vi "LED flashing 2.vi"(0 "Arduino Resource In":T1={"VISA resource"="", "Board Type"=enum."Uno", "Connection Type"=enum."USB / Serial", "Bytes Per Packet (15)"=15}, 11 "Error In":errorcluster, 12 "Текущий раствор":i32) -> (1 "1":bool, 2 "2":bool, 3 "3":bool, 4 "Arduino Resource Out":T1={"VISA resource"="", "Board Type"=enum."Uno", "Connection Type"=enum."USB / Serial", "Bytes Per Packet (15)"=15}, 15 "Error Out":errorcluster)   [LabVIEW 2016]
uses:
  <vilib>/LabVIEW Interface for Arduino/Type Defs/Arduino Resource.ctl
  <vilib>/LabVIEW Interface for Arduino/Type Defs/Board Type.ctl
  <vilib>/LabVIEW Interface for Arduino/LabVIEW Interface for Arduino.lvlib
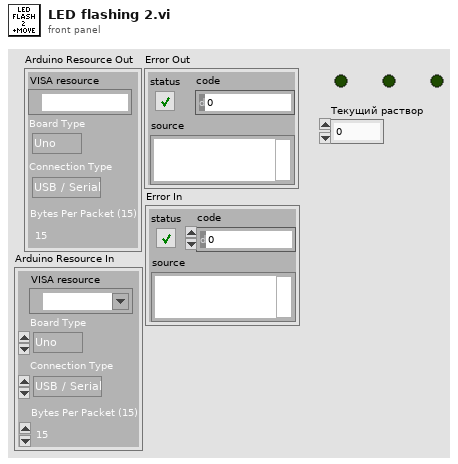
[diagram p1: front panel]
types:
  T1 = typedef "LabVIEW Interface for Arduino.lvlib/Arduino Resource.ctl" = cluster{"VISA resource":refnum<visa-resource-name>, "Board Type":T2, "Connection Type":enum8{"USB / Serial"}, "Bytes Per Packet (15)":u8}
  T2 = typedef "LabVIEW Interface for Arduino.lvlib/Board Type.ctl" = enum16{"Uno", "Dimuelanove w/Atmega 328", "Mega 2560"}
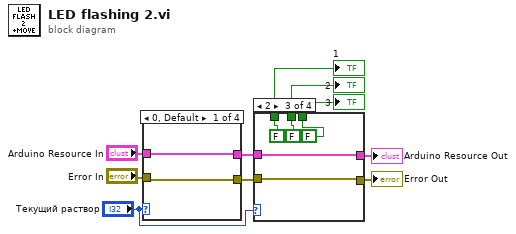
[diagram p0: block diagram]
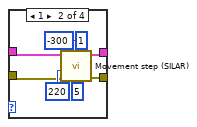
[diagram p2: hidden frame]
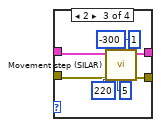
[diagram p3: hidden frame]
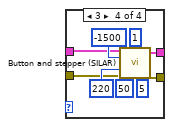
[diagram p4: hidden frame]
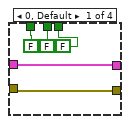
[diagram p5: hidden frame]
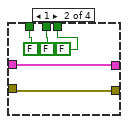
[diagram p6: hidden frame]
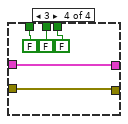
[diagram p7: hidden frame]
diagram:
  n1 = case shown="0, Default" "Текущий раствор" {
    tunnel: "Error In" -> [w12 w13 w21 w29]
    tunnel: [w11 w15 w23 w32] -> w3
    tunnel: [w12 w16 w24 w31] -> w4
    tunnel: "Arduino Resource In" -> [w11 w14 w22 w30]
    frame 0, Default {
    }
    frame 1 {
      n2 = call "Movement step (SILAR).vi"("ENABLE контакт"=u8 5 ("ENABLE Pin"), "Шаговый двигатель №"=u8 1 ("Stepper #"), "Error In"=w13, "Скорость"=i16 220 ("Set Speed (Steps per Second)"), "Кол-во шагов"=i16 -300 ("# of Steps to Move"), "Arduino Resource In"=w14) -> ("Error Out"=w16:errorcluster, "Arduino Resource Out"=w15:T1)  [unwired: 4 in]
    }
    frame 2 {
      n3 = call "Movement step (SILAR).vi"("ENABLE контакт"=u8 5 ("ENABLE Pin"), "Шаговый двигатель №"=u8 1 ("Stepper #"), "Error In"=w21, "Скорость"=i16 220 ("Set Speed (Steps per Second)"), "Кол-во шагов"=i16 -300 ("# of Steps to Move"), "Arduino Resource In"=w22) -> ("Error Out"=w24:errorcluster, "Arduino Resource Out"=w23:T1)  [unwired: 4 in]
    }
    frame 3 {
      n4 = call "Button and stepper (SILAR).vi"("Arduino Resource In"=w30, "Шаговый двигатель №"=u8 1 ("Stepper #"), "Кол-во шагов"=i16 -1500 ("# of Steps to Move"), "Скорость двигателя"=i16 220 ("Set Speed (Steps per Second)"), "Error In"=w29, "Контакт концевика"=u8 50 ("Digital I/O Pin (0)"), "ENABLE контакт"=u8 5 ("ENABLE Pin")) -> ("Arduino Resource Out"=w32:T1, "Error Out"=w31:errorcluster)  [unwired: 7 in]
    }
  }
  n5 = case shown="2" "Текущий раствор" {
    tunnel: w4 -> [w42 w43 w48 w53]
    tunnel: [w41 w44 w49 w54] -> w2
    tunnel: [w42 w43 w48 w53] -> w1
    tunnel: [FALSE ("3") FALSE ("3") FALSE ("3") FALSE ("3")] -> w10
    tunnel: [FALSE ("3") FALSE ("3") FALSE ("3") FALSE ("3")] -> w9
    tunnel: w3 -> [w41 w44 w49 w54]
    tunnel: [FALSE ("3") FALSE ("3") FALSE ("3") FALSE ("3")] -> w8
    frame 0, Default {
    }
    frame 1 {
    }
    frame 2 {
    }
    frame 3 {
    }
  }
  "1" <- w10
  "2" <- w8
  "3" <- w9
  "Arduino Resource Out" <- w2
  "Error Out" <- w1
